vi "add_quaternion.vi"(4 "Quaternion":cluster{"x":dbl, "y":dbl, "z":dbl, "w":dbl}, 5 "msg in":string) -> (2 "msg out":string)   [LabVIEW 2010]
uses:
  std_msgs/subs/float64Scalar.vi
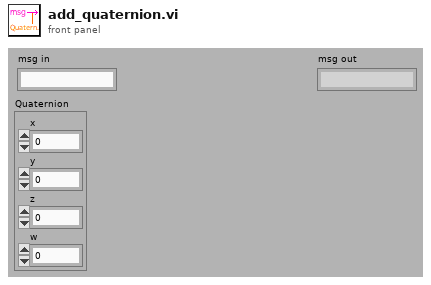
[diagram p1: front panel]
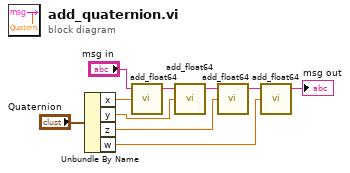
[diagram p0: block diagram]
diagram:
  n1 = Unbundle By Name("Quaternion") -> ("x"=w6:dbl, "y"=w5:dbl, "z"=w4:dbl, "w"=w3:dbl)
  n2 = call-poly "add_float64.vi"("Numeric"=w6, "msg in"="msg in") -> ("msg out"=w9:string)  [unwired: 3 in]
  n3 = call-poly "add_float64.vi"("Numeric"=w5, "msg in"=w9) -> ("msg out"=w8:string)  [unwired: 3 in]
  n4 = call-poly "add_float64.vi"("Numeric"=w4, "msg in"=w8) -> ("msg out"=w7:string)  [unwired: 3 in]
  n5 = call-poly "add_float64.vi"("Numeric"=w3, "msg in"=w7) -> ("msg out"=→"msg out":string)  [unwired: 3 in]
